vi "Test_Observe_ViewModelPublication_OK.vi"(8 "error in (no error)":errorcluster, 11 "TestObservation In":refnum<class "TestObservation.lvclass">) -> (0 "error out":errorcluster, 3 "TestObservation Out":refnum<class "TestObservation.lvclass">)   [LabVIEW 2017, in "TestPubSubRouting.lvlib" / "TestObservation.lvclass"]
uses:
  TestObservation.lvclass
  Source/Framework/Mediator/Mediator/Mediator.lvclass
  C:/Git/mva-framework/Source/Framework/IMediator/IMediator/IMediator.lvclass
  PublishingViewModel/PublishingViewModel.lvclass
  C:/Git/mva-framework/Source/Framework/IObserver/IObserver/IObserver.lvclass
  C:/Git/mva-framework/Source/Framework/IViewModel/IViewModel/IViewModel.lvclass
  C:/Program Files (x86)/National Instruments/LabVIEW 2017/vi.lib/ActorFramework/Actor/Actor.lvclass
  Source/Framework/IObserver/IObserver/IObserver.lvclass/IObserver.ctl
  Source/Framework/IMediator/IMediator/IMediator.lvclass/IMediator.ctl
  Source/Framework/IViewModel/IViewModel/IViewModel.lvclass/IViewModel.ctl
  Source/Framework/IViewManager/IViewManager Messages/Launch Nested Views Msg/Launch Nested Views Msg.lvclass/Launch Nested Views Msg.ctl
  Source/Framework/IViewManager/IViewManager/IViewManager.lvclass/IViewManager.ctl
  <vilib>/ActorFramework/Message Enqueuer/Message Enqueuer.lvclass/Message Enqueuer.ctl
  eb12c776-8aa7-441a-8f42-7366b3e7a185.vi
  Source/Framework/IObserver/IObserver/Configure Observer Logging.vi
  Source/Framework/IViewModel/IViewModel/Write Startup Model-View Configuration.vi
  Source/Framework/IMediator/IMediator/Configure Mediator.vi
  <vilib>/ActorFramework/Message Enqueuer/Enqueue.vi
  Source/Framework/IViewManager/IViewManager Messages/Launch Nested Views Msg/Pack Launch Nested Views Msg.vi
  Source/Framework/IViewManager/IViewManager/Write Startup Launch Nested Views Msg.vi
  ObservingModel/ObservingModel.lvclass
  C:/Git/mva-framework/Source/Framework/IModel/IModel/IModel.lvclass
  ObservingViewable/ObservingViewable.lvclass
  C:/Git/mva-framework/Source/Framework/IViewable/IViewable/IViewable.lvclass
  Source/Framework/IViewModel/IViewModel/IViewModel.lvclass
  C:/Git/mva-framework/Source/Framework/IViewManager/IViewManager/IViewManager.lvclass
  <vilib>/ActorFramework/Stop Msg/Stop Msg.lvclass
  C:/Program Files (x86)/National Instruments/LabVIEW 2017/vi.lib/ActorFramework/Message/Message.lvclass
  <vilib>/ActorFramework/Message Priority Queue/Priority Enqueue.vi
  gpm_packages/@cs/event-logger/Source/Composed Log/LoggerReference/LoggerReference.lvclass
  Source/Framework/IMediator/IMediatorBusMonitor/MediatorBusMonitor/IMediatorBusMonitor.lvclass
  gpm_packages/@cs/event-logger/Source/Text File Sink/Text File Sink.lvclass
  Source/Framework/IViewable/IApplicationStyle/IApplicationStyle.lvclass
  Source/Framework/IViewManager/IViewManager Messages/Launch Nested Views Msg/Launch Nested Views Msg.lvclass
  <vilib>/ActorFramework/Actor/Actor.lvclass
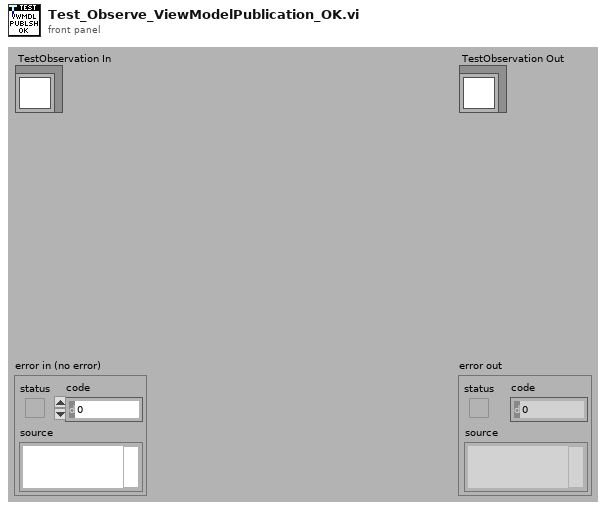
[diagram p1: front panel]
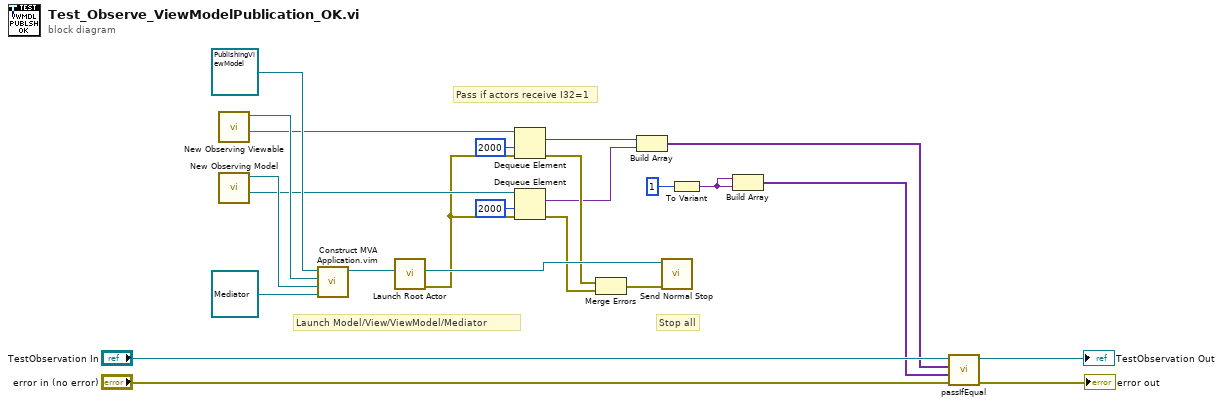
[diagram p0: block diagram]
diagram:
  # "Stop all"
  # "Launch Model/View/ViewModel/Mediator"
  # "Pass if actors receive I32=1"
  n1 = call "New Observing Viewable.vi"() -> ("Test Reply Queue"=w16:refnum<queue>, "ObservingViewable out"=w17:refnum<class "ObservingViewable.lvclass">)  [unwired: 10 in]
  n2 = call "New Observing Model.vi"() -> ("Test Reply Queue"=w9:refnum<queue>, "ObservingModel Out"=w11:refnum<class "ObservingModel.lvclass">)  [unwired: 10 in]
  n3 = call "Construct MVA Application.vim"("Mediator Type"=refnum<class "Mediator.lvclass"> refnum ("Mediator.lvlib:Mediator.lvclass"), "Model Type"=w11, "Startup View Configuration"=w17, "IViewModel In"=refnum<class "PublishingViewModel.lvclass"> refnum ("PublishingViewModel.lvclass")) -> ("IViewModel Out"=w18:refnum<class "PublishingViewModel.lvclass">)  [unwired: 7 in]
  n4 = call <vilib>:"Launch Root Actor.vi"("Actor"=w18) -> ("error out"=w5:errorcluster, "Actor's Enqueuer"=w14:refnum<class "Message Enqueuer.lvclass">)  [unwired: 9 in]
  n5 = Dequeue Element(queue=w16, timeout in ms (-1)=2000, error in (no error)=w5) -> (element=w13:variant, error out=w6:errorcluster)  [unwired: 2 out]
  n6 = Dequeue Element(queue=w9, timeout in ms (-1)=2000, error in (no error)=w5) -> (element=w3:variant, error out=w8:errorcluster)  [unwired: 2 out]
  n7 = Merge Errors(w6, w8) -> (w7:errorcluster)
  n8 = Build Array(w13, w3) -> (w4:variant[])
  n9 = call <vilib>:"Send Normal Stop.vi"("error in (no error)"=w7, "Message Enqueuer"=w14) -> ()  [unwired: 9 in, 1 out]
  n10 = To Variant(anything=1) -> (Variant=w1:variant)
  n11 = Build Array(w1, w1) -> (w2:variant[])
  n12 = call-dynamic "passIfEqual.vi"("error in (no error)"="error in (no error)", "y"=w2, "x"=w4, "TestCase in"="TestObservation In") -> ("error out"=→"error out":errorcluster, "TestCase out"=→"TestObservation Out":refnum<class "TestObservation.lvclass">)  [unwired: 6 in]
